vi "Execute.vi"(8 "error in (no error)":errorcluster, 11 "CIFPlugin in":refnum<class "Template_Plugin.lvclass">) -> (0 "error out":errorcluster, 3 "CIFPlugin out":refnum<class "Template_Plugin.lvclass">)   [LabVIEW 2021, in "Template_Plugin.lvclass"]
uses:
  Template_Plugin.lvclass
  C:/Program Files/National Instruments/LabVIEW 2021/vi.lib/CIF Foundation/CIF Core/CIFCore/Class/CIFCorePlugin.lvclass
  <vilib>/CIF Foundation/CIF Core/CIFCore/Class/Typedef/Energized States.ctl
  <vilib>/CIF Foundation/CIF Core/CIFCore/Class/CIFCorePlugin.lvclass/CIFCorePlugin.ctl
  <vilib>/CIF Foundation/CIF Core/CIFCore/Class/Accessors/Timestamps/Write Execute TS.vi
  <vilib>/CIF Foundation/CIF Core/CIFCore/Class/Accessors/Timestamps/Write Sleep TS.vi
  <vilib>/Utility/error.llb/Clear Errors.vi
  <vilib>/CIF Foundation/CIF Utilities/Time/System Time/Sleep Until Future Time.vi
  <vilib>/CIF Foundation/CIF Core/CIFCore/Class/Accessors/Read Sleep Limits (ns).vi
  <vilib>/CIF Foundation/CIF Core/CIFCore/Class/Accessors/Timestamps/Write Target Wake TS.vi
  <vilib>/CIF Foundation/CIF Core/CIFCore/Class/SubVIs/Start Running.vi
  <vilib>/CIF Foundation/CIF Core/CIFCore/Class/Accessors/Read Plugin Name.vi
  <vilib>/CIF Foundation/CIF Utilities/Time/System Time/Get System Time.vi
  <vilib>/CIF Foundation/CIF Core/CIFCore/Common/Utilities/Add Error.vi
  <vilib>/CIF Foundation/CIF Core/CIFCore/Class/Accessors/Timestamps/Read Running TS.vi
  <vilib>/CIF Foundation/CIF Core/CIFCore/Class/Benchmarking/Reset Delay.vi
  <vilib>/CIF Foundation/CIF Core/CIFCore/Class/Accessors/Read Running Internal Data.vi
  <vilib>/CIF Foundation/CIF Core/CIFCore/Class/Accessors/Read Timing Override.vi
  <vilib>/CIF Foundation/CIF Core/CIFCore/Class/Accessors/Read Common Config.vi
  <vilib>/CIF Foundation/CIF Utilities/Time/SubVIs/Add Error.vi
  <vilib>/CIF Foundation/CIF Utilities/Time/System Time/LabVIEW Time to TAI Time.vi
  <vilib>/CIF Foundation/CIF Utilities/Errors/Append Error Location.vi
  Template_Plugin.lvclass/Template_Plugin.ctl
  <vilib>/CIF Foundation/CIF Core/CIFCore/Class/CIFCorePlugin.lvclass
  D:/dev/Plugins/Template/src/Template/Class/Template_Plugin.lvclass
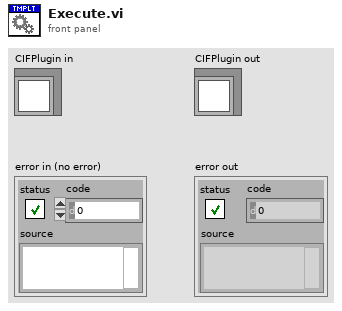
[diagram p1: front panel]
types:
  T1 = typedef "CIFCorePlugin.lvclass/Energized States.ctl" = enum16{"Listen", "Prepare", "Execute", "Housekeep", "Cleanup", "Destroy"}
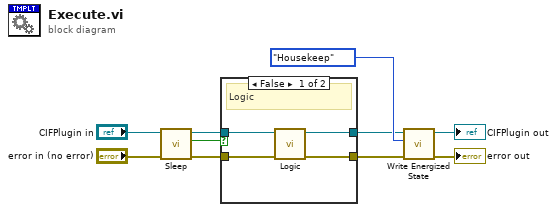
[diagram p0: block diagram]
diagram:
  n1 = call <vilib>:"Sleep.vi"("error in (no error)"="error in (no error)", "CIFCorePlugin in"="CIFPlugin in") -> ("error out"=w7:errorcluster, "Housekeep only"=w8:bool, "CIFCorePlugin out"=w6:refnum<class "Template_Plugin.lvclass">)  [unwired: 7 in]
  n2 = case shown="False" w8 {
    tunnel: [w12 w15] -> w1
    tunnel: [w13 w16] -> w9
    tunnel: w6 -> [w14 w16]
    tunnel: w7 -> [w11 w15]
    frame False {
      # "Logic"
      n3 = call "Logic.vi"("error in (no error)"=w11, "CIFPlugin in"=w14) -> ("error out"=w12:errorcluster, "CIFPlugin out"=w13:refnum<class "Template_Plugin.lvclass">)  [unwired: 8 in]
    }
    frame True {
      # "Housekeep only"
    }
  }
  n4 = call <vilib>:"Write Energized State.vi"("error in (no error)"=w1, "Energized State"=Energized_States."Housekeep", "CIFCorePlugin in"=w9) -> ("error out"=→"error out":errorcluster, "CIFCorePlugin out"=→"CIFPlugin out":refnum<class "Template_Plugin.lvclass">)  [unwired: 7 in]
